vi "API_DB.UpdateInventoryRecord.vi"(0 "Database in":refnum<class "Database.lvclass">, 1 "Wait (F)":bool, 2 "InventoryRecord.Location.Module":u16, 3 "InventoryRecord.LocationStatus":T1, 5 "Record.ReticleID":string, 7 "InventoryRecord.Stocker":T2 items=["Main", "Exp1", "Exp2"], 9 "Table":string, 11 "error in (no error)":errorcluster, 12 "Timeout (ms)":u32, 13 "InventoryRecord.Location.Row":u16, 14 "InventoryRecord.Location.Column":u16) -> (4 "Database out":refnum<class "Database.lvclass">, 6 "Slot":string, 15 "error out":errorcluster)   [LabVIEW 2020, in "Database.lvclass"]
doc: "Developed by Kevin Thompson\nkevin@thompsonengineering.net\n\nCopyright 2018\nThompson Engineering, LLC"
uses:
  Database.lvclass
  DataTypes/Stocker--Enum.ctl
  DataTypes/LocationStatus--Enum.ctl
  DataTypes/AsynCmd_Temp01--enum.ctl
  DataTypes/GenericQuery--Cluster.ctl
  DataTypes/SQLQuery--Enum.ctl
  DataTypes/InventoryRecord--Cluster.ctl
  DataTypes/Module--Cluster.ctl
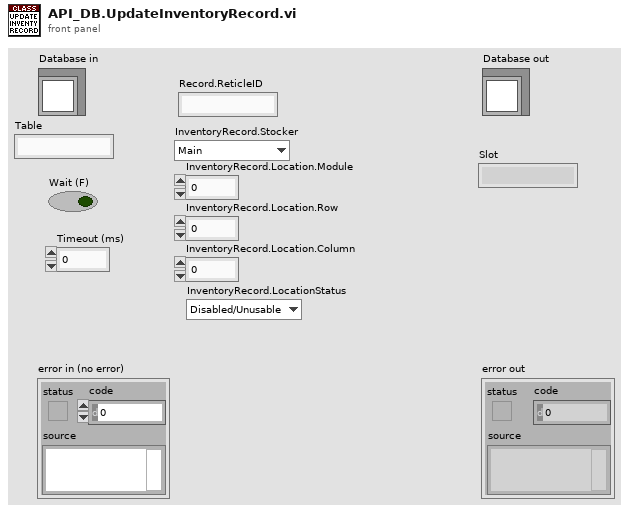
[diagram p1: front panel]
types:
  T1 = typedef "LocationStatus--Enum.ctl" = enum16{"Disabled/Unusable", "Full", "Empty"}
  T2 = typedef "Stocker--Enum.ctl" = u16
  T3 = typedef "SQLQuery--Enum.ctl" = enum16{"GetInventoryRecordFromDB", "GetReticleInfoFromDB", "GetLocationStatusFromDB", "UpdateInventoryRecord", "UpdateLocationStatus", "UpdateReticleLocationStatus", "AddReticleInDB", "RemoveReticleAtLocation", "RemoveReticleUsingReticleID", "GetLocationForReticleID", "GetAllLocations", "GetAllEmptyLocations", "GetAllLocationsInStocker", "GetAllFullLocations", "GetAllFullLocationsInStocker", "GetAllDisabledLocations", "GetAllDisabledLocationsInStocker", "FindFirstSlot"}
  T4 = typedef "GenericQuery--Cluster.ctl" = cluster{"Query":T3, "Table":string, "InventoryRecord":T5}
  T5 = typedef "InventoryRecord--Cluster.ctl" = cluster{"ReticleID":string, "Stocker":T2, "Location":T6, "LocationStatus":T1, "EquipmentID":string, "LocationID":string}
  T6 = typedef "Module--Cluster.ctl" = cluster{"Module":u16, "Row":u16, "Column":u16}
  T7 = typedef "Database.lvclass/AsynCmd_Temp01--enum.ctl" = enum16{"DB.DeleteRecord", "DB.UpdateRecord", "DB.InsertRecord", "DB.SelectRecord", "DB.ExecuteSQLCommand", "DB.FindFirstSlot", "DB.GenericSQLQuery"}
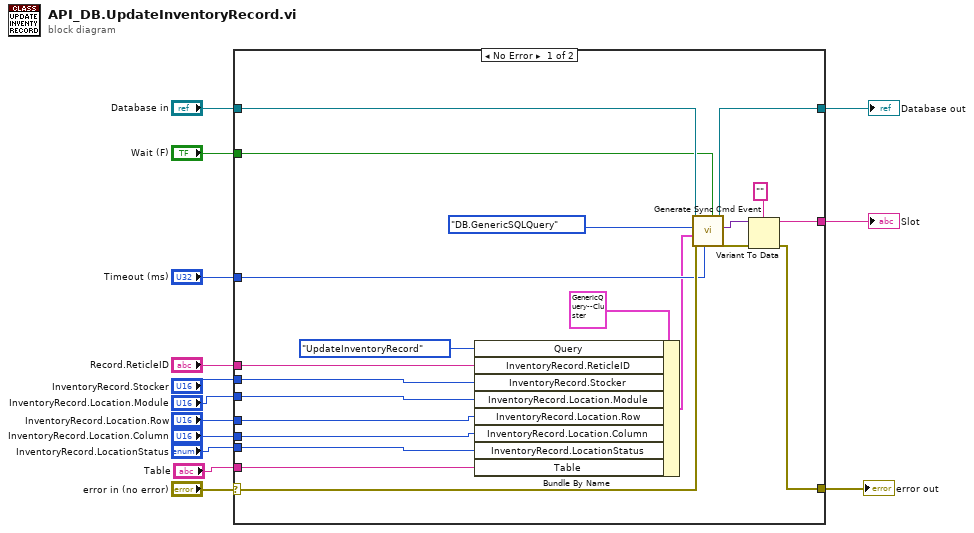
[diagram p0: block diagram]
diagram:
  n1 = case shown="No Error" "error in (no error)" {
    selector: "error in (no error)" -> [w33 w37]
    tunnel: [w28 w37] -> w13
    tunnel: [w34 w36] -> w11
    tunnel: "Database in" -> [w35 w36]
    tunnel: [w30 _] -> w8
    tunnel: "Wait (F)" -> [w27 _]
    tunnel: "Timeout (ms)" -> [w26 _]
    tunnel: "Record.ReticleID" -> [w21 _]
    tunnel: "InventoryRecord.Stocker" -> [w20 _]
    tunnel: "InventoryRecord.Location.Module" -> [w19 _]
    tunnel: "InventoryRecord.Location.Row" -> [w18 _]
    tunnel: "InventoryRecord.Location.Column" -> [w17 _]
    tunnel: "InventoryRecord.LocationStatus" -> [w16 _]
    tunnel: "Table" -> [w15 _]
    frame No Error {
      n2 = Bundle By Name(cluster=T4 {"Query"=enum."GetInventoryRecordFromDB", "Table"="", "InventoryRecord"={"ReticleID"="", "Stocker"=0, "Location"={"Module"=0, "Row"=0, "Column"=0}, "LocationStatus"=enum."Disabled/Unusable", "EquipmentID"="", "LocationID"=""}}, "Query"=SQLQuery--Enum."UpdateInventoryRecord", "InventoryRecord.ReticleID"=w21, "InventoryRecord.Stocker"=w20, "InventoryRecord.Location.Module"=w19, "InventoryRecord.Location.Row"=w18, "InventoryRecord.Location.Column"=w17, "InventoryRecord.LocationStatus"=w16, "Table"=w15) -> (w22:T4)
      n3 = call "Generate Sync Cmd Event.vi"("Wait (F)"=w27, "Timeout (ms)"=w26, "error in (no error)"=w33, "vData"=w22, "AsyncCmd"=AsynCmd_Temp01--enum."DB.GenericSQLQuery", "Database in"=w35) -> ("error out"=w29:errorcluster, "Return Value"=w31:variant, "Database out"=w34:refnum<class "Database.lvclass">)  [unwired: 3 in]
      n4 = Variant To Data(error in=w29, type="", Variant=w31) -> (data=w30:string, error out=w28:errorcluster)
    }
    frame Error {
    }
  }
  "error out" <- w13
  "Database out" <- w11
  "Slot" <- w8
